vi "test.StateIterator_Advance.vi"() -> ()   [LabVIEW 2017]
uses:
  cda3732c-20de-4d78-8484-3f83ac87b9b8.vi
  cda3732c-20de-4d78-8484-3f83ac87b9b8.vi/f32593b9-91d5-444e-80f1-1e5e2bced81b.vi
  <userlib>/_OpenG.lib/lvdata/lvdata.llb/Get Strings from Enum__ogtk.vi
  b488c091-78ba-40d2-ac7d-d3a4231e3f9a.vi
  9db92dec-6ee7-4ae5-a3b3-7eb4b823bb0d.vi
panel:
  out "String":string
  in  "stop":bool
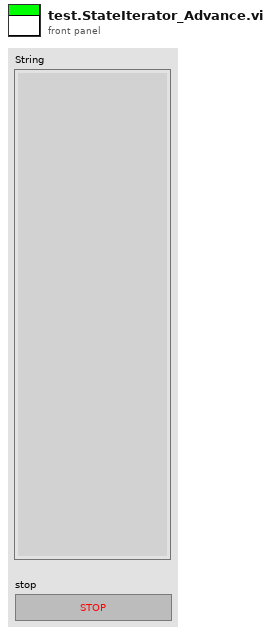
[diagram p1: front panel]
types:
  T1 = enum16{"0", "1", "2", "3", "4", "5", "6", "7", "8", "9"}
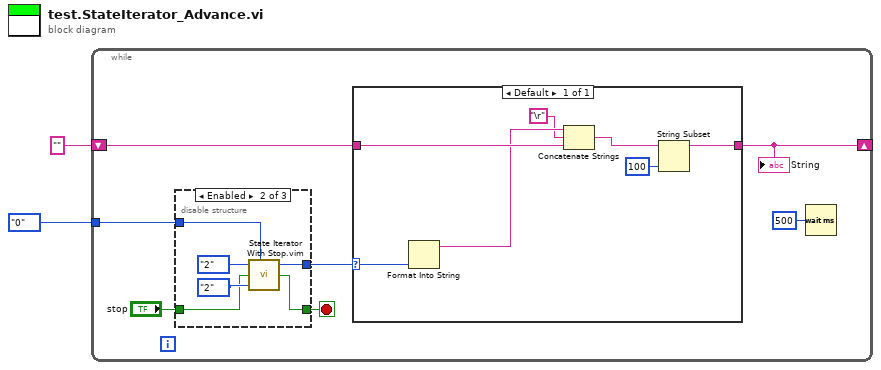
[diagram p0: block diagram]
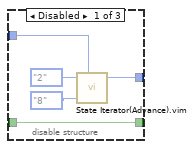
[diagram p2: hidden frame]
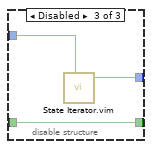
[diagram p3: hidden frame]
diagram:
  n1 = while {
    tunnel: T1."0" -> [w9]
    shift-right: [w6] -> _
    shift-left: "" -> [w7]
    stop <- w3 stop-if-true
    n2 = disable-structure shown="Enabled" {
      disable-tunnel: w9 -> [w14 w20 w22]
      disable-tunnel: [w13 w19 w23] -> w8
      disable-tunnel: "stop" -> [w10 w16 w21]
      disable-tunnel: [w10 w15 w21] -> w3
      frame Disabled {
        n3 = call "State Iterator(Advance).vim"("Start State"=T1."2", "SM Typedef"=w14, "End State"=T1."8") -> ("State"=w13:T1)  [unwired: 4 in]
      }
      frame Enabled {
        n4 = call "State Iterator With Stop.vim"("Start State"=T1."2", "SM Typedef"=w20, "Stop?"=w16, "End State"=T1."2") -> ("State"=w19:T1, "Terminal Loop?"=w15:bool)  [unwired: 2 in]
      }
      frame Disabled {
        n5 = call "State Iterator.vim"("StateMachine Typedef"=w22) -> ("State"=w23:T1)  [unwired: 6 in]
      }
    }
    n6 = case shown="Default" w8 {
      selector: w8 -> [w30]
      tunnel: w7 -> [w29]
      tunnel: [w25] -> w6
      frame Default {
        n7 = Format Into String(w30) -> (resulting string=w27:string)  [unwired: 3 in, 1 out]
        n8 = Concatenate Strings(w27, "\r", w29) -> (w28:string)
        n9 = String Subset(string=w28, length (rest)=100 ("length (rest)")) -> (substring=w25:string)  [unwired: 1 in]
      }
    }
    "String" <- w6
    n10 = Wait (ms)(milliseconds to wait=u32 500) -> ()  [unwired: 1 out]
  }
